vi "Get_NodeValue.vi"(8 "error in":errorcluster, 10 "node name":string, 11 "node in":refnum<k20>) -> (0 "error out":errorcluster, 1 "NotFound":bool, 2 "node text":string, 3 "node out":refnum<k20>)   [LabVIEW 2010, in "Pansino_XML_Read.lvlib"]
uses:
  <vilib>/xml/Close Reference(Node).vi
  Pansino_XML_Read.lvlib
  <vilib>/xml/NI_XML.lvlib
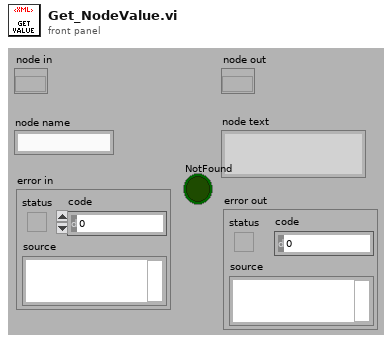
[diagram p1: front panel]
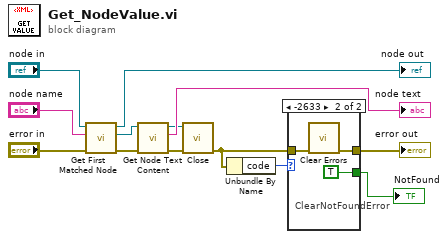
[diagram p0: block diagram]
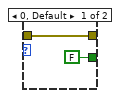
[diagram p2: hidden frame]
diagram:
  n1 = call <vilib>:"Get First Matched Node.vi"("error in (no error)"="error in", "XPath expression"="node name", "node in"="node in") -> ("error out"=w9:errorcluster, "node result"=w6:refnum<k20>, "node out"=→"node out":refnum<k20>)  [unwired: 6 in]
  n2 = call <vilib>:"Get Node Text Content.vi"("error in (no error)"=w9, "node in"=w6) -> ("error out"=w12:errorcluster, "node text"=→"node text":string, "node out"=w11:refnum<k20>)  [unwired: 7 in]
  n3 = call-poly <vilib>:"Close.vi"("error in (no error)"=w12, "node"=w11) -> ("error out"=w3:errorcluster)  [unwired: 7 out]
  n4 = Unbundle By Name(w3) -> ("code"=w4:i32)
  n5 = case shown="-2633" w4 {
    tunnel: w3 -> [w15 w18]
    tunnel: [w15 w17] -> w2
    tunnel: [FALSE TRUE] -> w1
    frame 0, Default {
    }
    frame -2633 {
      # "ClearNotFoundError"
      n6 = call <vilib>:"Clear Errors.vi"("error in (no error)"=w18) -> ("error out"=w17:errorcluster)  [unwired: 6 in]
    }
  }
  "error out" <- w2
  "NotFound" <- w1
